vi "Configuration to String.vi"(8 "error in (no error)":errorcluster, 10 "Configuration":variant, 11 "Instrument":T2=enum."Switching Matrix") -> (0 "error out":errorcluster, 2 "Instrument Configuration":T1={"Instrument"=enum."Switching Matrix", "Configuration"="Test Configuration"})   [LabVIEW 2014]
uses:
  Measurements/Instrument Sequence/Hardware Configuration.ctl
  Hardware Control/Spectrometer/Spectrometer Config.ctl
  Hardware Control/Spectrometer/Laser Settings.ctl
  Hardware Control/Spectrometer/Laser.ctl
  Hardware Control/Spectrometer/Filter.ctl
  Hardware Control/Spectrometer/Grating Detector Settings.ctl
  Hardware Control/Spectrometer/Grating.ctl
  Hardware Control/Spectrometer/Detector.ctl
  Hardware Control/Spectrometer/Acquisition Settings.ctl
  Hardware Control/Switches and Mirrors/SwitchesMirrors Config.ctl
  Hardware Control/Switches and Mirrors/SwitchesMirrors Status.ctl
  Hardware Control/Stress Control/StressControl Config.ctl
  Hardware Control/Parameter Analyzer/Parameter Analyzer Config.ctl
  Hardware Control/Parameter Analyzer/Parameter Analyzer Integration Parameters.ctl
  Hardware Control/Parameter Analyzer/Parameter Analyzer SMU Sweeping.ctl
  Hardware Control/Parameter Analyzer/Parameter Analyzer Sweep Spacing.ctl
  Hardware Control/Parameter Analyzer/Parameter Analyzer SMU Range.ctl
  Hardware Control/Parameter Analyzer/Parameter Analyzer SMU Sampling.ctl
  Hardware Control/Parameter Analyzer/Parameter Analyzer Sampling Parameters.ctl
  Hardware Control/Parameter Analyzer/Parameter Analyzer Stop Sampling Conditions.ctl
  Hardware Control/Switching Matrix/Switching Matrix Config.ctl
  Measurements/Save Data/SaveData Workspace Info.ctl
  Measurements/Instrument Sequence/Instrument List.ctl
  Measurements/Save Data/SaveData Instrument Configuration.ctl
panel:
  in  "Hardware Configuration":T3={"Optical Spectrometer"={"Laser Settings"={"Laser Wavelength"=enum."784 nm", "Neutral Density Filter"=enum."50%"}, "Spectrometer Settings"={"Confocal Hole Size (µm)"=150.0, "Grating"=2, "Detector"=enum."InGaAs Array"}, "Acquisition Settings"={"Acquisition Mode"=enum."Single Window", "Spectal Position (nm)"=632.84, "From (nm)"=632.84, "To (nm)"=1.0, "Integration Time (s)"=3.0, "Number of Accumulations"=3, "AutoScanning"=FALSE, "Spike Removal"=FALSE}, "Path"=path ""}, "Switches & Mirrors"={"Relay VISA Session"="COM1", "Switches"={"Laser"=FALSE, "Video"=FALSE}, "Delays (ms)"={"Laser"=500, "Video"=1500}}, "StressControl"={"Stress Control VISA Session"="COM4", "Axis"=1, "Motion"=0, "Destination (°)"=0.0, "Speed (°/s)"=4.0, "Position (°)"=0.0}, "Parameter Analizer"={"Parameter Analyzer VISA Session"="GPIB0::27::INSTR", "Sweeping Time Parameters"={"Integration Time"=0, "Short Integration Time (s)"=0.00192, "Long Integration Time (s)"=0.02, "Wait Time Parameter"=1.0}, "Acquisition Mode"=enum."Sweeping Mode", "Status Polling Time (ms)"=1000, "Comment"="", "SMU 1 - Sweeping"={"Start / Offset"=0.0, "Stop / Ratio"=10.0, "Step \n(linear only)"=0.01, "Compliance"=0.1, "Power \nCompliance"=0.0, "Mode"=0, "Function"=1, "Sweep Mode"=FALSE}, "SMU 2 - Sweeping"={"Start / Offset"=0.0, "Stop / Ratio"=1.0, "Step \n(linear only)"=0.01, "Compliance"=10.0, "Power \nCompliance"=0.0, "Mode"=1, "Function"=4, "Sweep Mode"=FALSE}, "SMU 3 - Sweeping"={"Start / Offset"=0.0, "Stop / Ratio"=1.0, "Step \n(linear only)"=0.01, "Compliance"=10.0, "Power \nCompliance"=0.0, "Mode"=1, "Function"=4, "Sweep Mode"=FALSE}, "SMU 4 - Sweeping"={"Start / Offset"=0.0, "Stop / Ratio"=1.0, "Step \n(linear only)"=0.01, "Compliance"=0.1, "Power \nCompliance"=0.0, "Mode"=0, "Function"=4, "Sweep Mode"=FALSE}, "Sweep Spacing"=0, "Range"=0, "SMU1 - Sampling"={"Source"=10.0, "Compliance"=0.01, "Mode"=0, "Function"=FALSE}, "SMU2 - Sampling"={"Source"=0.0, "Compliance"=10.0, "Mode"=1, "Function"=FALSE}, "SMU3 - Sampling"={"Source"=0.0, "Compliance"=10.0, "Mode"=1, "Function"=FALSE}, "SMU4 - Sampling"={"Source"=0.0, "Compliance"=0.01, "Mode"=0, "Function"=FALSE}, "Sampling Time Parameters"={"Initial Interval (s)"=0.1, "Number of Samples"=60, "Total Sampling Time (s)"=10.0, "Hold Time (s)"=0.0, "Sampling Mode"=0, "Sampling Time"=0}, "Stop Condition"={"Enable Delay (s)"=0.0, "Name"="", "Threshold"=0.0, "num. of events"=1, "Event"=0, "Stop Condition Enable"=FALSE}}, "Switching Matrix"={"Switching Matrix VISA Session"="GPIB0::18::INSTR", "Connections"=[{"Connections"=[TRUE, FALSE, FALSE, FALSE, FALSE, FALSE, FALSE, FALSE, FALSE, FALSE, FALSE, FALSE], "Connection Type"=enum."Make - Break"}, {"Connections"=[FALSE, TRUE, FALSE, FALSE, FALSE, FALSE, FALSE, FALSE, FALSE, FALSE, FALSE, FALSE], "Connection Type"=enum."Make - Break"}, {"Connections"=[FALSE, FALSE, TRUE, FALSE, FALSE, FALSE, FALSE, FALSE, FALSE, FALSE, FALSE, FALSE], "Connection Type"=enum."Make - Break"}, {"Connections"=[FALSE, FALSE, FALSE, TRUE, FALSE, FALSE, FALSE, FALSE, FALSE, FALSE, FALSE, FALSE], "Connection Type"=enum."Make - Break"}, {"Connections"=[FALSE, FALSE, FALSE, FALSE, TRUE, TRUE, TRUE, TRUE, TRUE, TRUE, TRUE, TRUE], "Connection Type"=enum."Make - Break"}, {"Connections"=[FALSE, FALSE, FALSE, FALSE, FALSE, FALSE, FALSE, FALSE, FALSE, FALSE, FALSE, FALSE], "Connection Type"=enum."Disconnected"}, {"Connections"=[FALSE, FALSE, FALSE, FALSE, FALSE, FALSE, FALSE, FALSE, FALSE, FALSE, FALSE, FALSE], "Connection Type"=enum."Disconnected"}, {"Connections"=[FALSE, FALSE, FALSE, FALSE, FALSE, FALSE, FALSE, FALSE, FALSE, FALSE, FALSE, FALSE], "Connection Type"=enum."Disconnected"}]}, "Electrical Measurement"={"Measurement Type"=enum."Four Probe", "Sweep Mode"=FALSE, "Force Mode"=enum."Voltage", "Maximum Force"=0.15, "Step Size"=0.001, "Compliance"=0.001, "Power Compliance"=0.0, "Integration Time (s)"=0.02}, "Workspace Info"={"Device Name"="test", "Device Info"="test", "Path"=path "C:/Users/gio/Desktop/test Python2Workspace/python2workspace_test.pmat"}, "AutoFocus Status"={"Update Refnums"=FALSE, "Allocate Image Memory"=FALSE, "Set Match Criteria"=FALSE, "Link Stage & Camera"=FALSE, "Set Target"=FALSE, "Find Target"=FALSE}} {"Electrical Measurement"."Integration Time (s)" min=0.02 max=2.0 scale=8e-05..2.0; "Electrical Measurement"."Power Compliance" format="%^.2e"; "Electrical Measurement"."Compliance" format="%^.2e"; "Electrical Measurement"."Step Size" format="%^.4e"; "Electrical Measurement"."Maximum Force" format="%^.4e"; "Parameter Analizer"."Stop Condition"."Event" items=["Value > Threshold", "Value < Threshold", "| Value | > | Threshold |", "| Value | < | Threshold |"]; "Parameter Analizer"."Stop Condition"."Threshold" format="%^.2e"; "Parameter Analizer"."Stop Condition"."Enable Delay (s)" format="%.1f"; "Parameter Analizer"."Sampling Time Parameters"."Sampling Time" items=["Auto (linear only)", "No Limit", "Set Limit"]; "Parameter Analizer"."Sampling Time Parameters"."Sampling Mode" items=["Linear", "Log10", "Log25", "Log50", "Thinned Out"]; "Parameter Analizer"."Sampling Time Parameters"."Hold Time (s)" format="%.4f"; "Parameter Analizer"."Sampling Time Parameters"."Total Sampling Time (s)" format="%.1f"; "Parameter Analizer"."Sampling Time Parameters"."Initial Interval (s)" format="%^.3e"; "Parameter Analizer"."SMU 4 - Sweeping"."Function" items=["Disabled", "Var 1", "Var 2", "Var 1'", "Constant"]; "Parameter Analizer"."SMU 4 - Sweeping"."Mode" items=["V", "I", "V pulse", "I  pulse", "Common"]; "Parameter Analizer"."SMU 4 - Sweeping"."Power \nCompliance" format="%^.2e"; "Parameter Analizer"."SMU 4 - Sweeping"."Compliance" format="%^.2e"; "Parameter Analizer"."SMU 4 - Sweeping"."Step \n(linear only)" format="%^.4e"; "Parameter Analizer"."SMU 4 - Sweeping"."Stop / Ratio" format="%^.4e"; "Parameter Analizer"."SMU 4 - Sweeping"."Start / Offset" format="%^.4e"; "Parameter Analizer"."SMU 3 - Sweeping"."Function" items=["Disabled", "Var 1", "Var 2", "Var 1'", "Constant"]; "Parameter Analizer"."SMU 3 - Sweeping"."Mode" items=["V", "I", "V pulse", "I  pulse", "Common"]; "Parameter Analizer"."SMU 3 - Sweeping"."Power \nCompliance" format="%^.2e"; "Parameter Analizer"."SMU 3 - Sweeping"."Compliance" format="%^.2e"; "Parameter Analizer"."SMU 3 - Sweeping"."Step \n(linear only)" format="%^.4e"; "Parameter Analizer"."SMU 3 - Sweeping"."Stop / Ratio" format="%^.4e"; "Parameter Analizer"."SMU 3 - Sweeping"."Start / Offset" format="%^.4e"; "Parameter Analizer"."SMU 2 - Sweeping"."Function" items=["Disabled", "Var 1", "Var 2", "Var 1'", "Constant"]; "Parameter Analizer"."SMU 2 - Sweeping"."Mode" items=["V", "I", "V pulse", "I  pulse", "Common"]; "Parameter Analizer"."SMU 2 - Sweeping"."Power \nCompliance" format="%^.2e"; "Parameter Analizer"."SMU 2 - Sweeping"."Compliance" format="%^.2e"; "Parameter Analizer"."SMU 2 - Sweeping"."Step \n(linear only)" format="%^.4e"; "Parameter Analizer"."SMU 2 - Sweeping"."Stop / Ratio" format="%^.4e"; "Parameter Analizer"."SMU 2 - Sweeping"."Start / Offset" format="%^.4e"; "Parameter Analizer"."SMU 1 - Sweeping"."Function" items=["Disabled", "Var 1", "Var 2", "Var 1'", "Constant"]; "Parameter Analizer"."SMU 1 - Sweeping"."Mode" items=["V", "I", "V pulse", "I  pulse", "Common"]; "Parameter Analizer"."SMU 1 - Sweeping"."Power \nCompliance" format="%^.2e"; "Parameter Analizer"."SMU 1 - Sweeping"."Compliance" format="%^.2e"; "Parameter Analizer"."SMU 1 - Sweeping"."Step \n(linear only)" format="%^.4e"; "Parameter Analizer"."SMU 1 - Sweeping"."Stop / Ratio" format="%^.4e"; "Parameter Analizer"."SMU 1 - Sweeping"."Start / Offset" format="%^.4e"; "Parameter Analizer"."Sweeping Time Parameters"."Long Integration Time (s)" scale=0.02..2.0; "Parameter Analizer"."Sweeping Time Parameters"."Short Integration Time (s)" scale=8e-05..0.00192; "Parameter Analizer"."Sweeping Time Parameters"."Integration Time" items=["Short", "Long"]; "Parameter Analizer"."Sweeping Time Parameters"."Wait Time Parameter" format="%.1f"; "Parameter Analizer"."SMU4 - Sampling"."Mode" items=["V", "I", "Common"]; "Parameter Analizer"."SMU4 - Sampling"."Compliance" format="%^.2e"; "Parameter Analizer"."SMU4 - Sampling"."Source" format="%^.3e"; "Parameter Analizer"."SMU3 - Sampling"."Mode" items=["V", "I", "Common"]; "Parameter Analizer"."SMU3 - Sampling"."Compliance" format="%^.2e"; "Parameter Analizer"."SMU3 - Sampling"."Source" format="%^.3e"; "Parameter Analizer"."SMU2 - Sampling"."Mode" items=["V", "I", "Common"]; "Parameter Analizer"."SMU2 - Sampling"."Compliance" format="%^.2e"; "Parameter Analizer"."SMU2 - Sampling"."Source" format="%^.3e"; "Parameter Analizer"."SMU1 - Sampling"."Mode" items=["V", "I", "Common"]; "Parameter Analizer"."SMU1 - Sampling"."Compliance" format="%^.2e"; "Parameter Analizer"."SMU1 - Sampling"."Source" format="%^.3e"; "Parameter Analizer"."Range" items=["auto", "fixed", "limited"]; "Parameter Analizer"."Sweep Spacing" items=["linear", "log 10", "log 25", "log 50"]; "StressControl"."Axis" min=1 max=3; "StressControl"."Position (°)" format="%.6g"; "StressControl"."Speed (°/s)" min=0.0 max=4.0 format="%.6f"; "StressControl"."Destination (°)" min=-2000000000.0 max=2000000000.0 format="%.6f"; "StressControl"."Motion" items=["Absolute", "Relative"]; "Optical Spectrometer"."Spectrometer Settings"."Grating" items=["1800 l/mm", "150 l/mm"]}
  # "LICENSED MATERIALS – PROPERTY OF IBM\nCopyright IBM Corp. 2016,\nALL RIGHTS RESERVED"
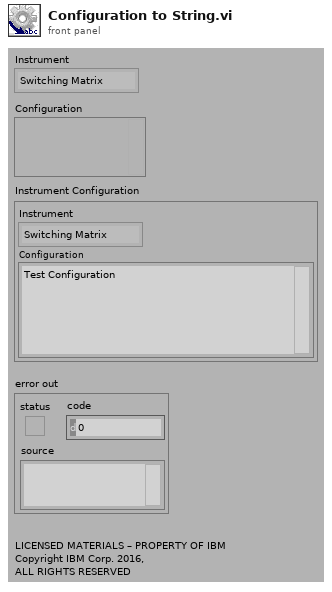
[diagram p1: front panel]
types:
  T1 = typedef "SaveData Instrument Configuration.ctl" = cluster{"Instrument":T2, "Configuration":string}
  T2 = typedef "Instrument List.ctl" = enum32{"Unknown Instrument", "Switching Matrix", "Parameter Analyzer", "Optical Spectrometer", "Optoelectronic", "Autofocus"}
  T3 = typedef "Hardware Configuration.ctl" = cluster{"Optical Spectrometer":T4, "Switches & Mirrors":T12, "StressControl":T14, "Parameter Analizer":T15, "Switching Matrix":T23, "Electrical Measurement":cluster{"Measurement Type":enum32{"Four Probe", "Two Probe"}, "Sweep Mode":bool, "Force Mode":enum32{"Voltage", "Current"}, "Maximum Force":dbl, "Step Size":dbl, "Compliance":dbl, "Power Compliance":dbl, "Integration Time (s)":dbl}, "Workspace Info":T24, "AutoFocus Status":cluster{"Update Refnums":bool, "Allocate Image Memory":bool, "Set Match Criteria":bool, "Link Stage & Camera":bool, "Set Target":bool, "Find Target":bool}}
  T4 = typedef "Spectrometer Config.ctl" = cluster{"Laser Settings":T5, "Spectrometer Settings":T8, "Acquisition Settings":T11, "Path":path}
  T5 = typedef "Laser Settings.ctl" = cluster{"Laser Wavelength":T6, "Neutral Density Filter":T7}
  T6 = typedef "Laser.ctl" = enum16{"633 nm", "784 nm", "532 nm", "365 nm"}
  T7 = typedef "Filter.ctl" = enum16{"100%", "50%", "25%", "10%", "1%", "0.1%", "0.01%"}
  T8 = typedef "Grating Detector Settings.ctl" = cluster{"Confocal Hole Size (µm)":dbl, "Grating":T9, "Detector":T10}
  T9 = typedef "Grating.ctl" = u16
  T10 = typedef "Detector.ctl" = enum16{"InGaAs Array", "Silicon CCD"}
  T11 = typedef "Acquisition Settings.ctl" = cluster{"Acquisition Mode":enum16{"Single Window", "Multi-Window"}, "Spectal Position (nm)":dbl, "From (nm)":dbl, "To (nm)":dbl, "Integration Time (s)":dbl, "Number of Accumulations":i32, "AutoScanning":bool, "Spike Removal":bool}
  T12 = typedef "SwitchesMirrors Config.ctl" = cluster{"Relay VISA Session":refnum<visa-resource-name>, "Switches":T13, "Delays (ms)":cluster{"Laser":u32, "Video":u32}}
  T13 = typedef "SwitchesMirrors Status.ctl" = cluster{"Laser":bool, "Video":bool}
  T14 = typedef "StressControl Config.ctl" = cluster{"Stress Control VISA Session":refnum<visa-resource-name>, "Axis":i32, "Motion":u16, "Destination (°)":dbl, "Speed (°/s)":dbl, "Position (°)":dbl}
  T15 = typedef "Parameter Analyzer Config.ctl" = cluster{"Parameter Analyzer VISA Session":refnum<visa-resource-name>, "Sweeping Time Parameters":T16, "Acquisition Mode":enum32{"Sweeping Mode", "Sampling Mode"}, "Status Polling Time (ms)":u32, "Comment":string, "SMU 1 - Sweeping":T17, "SMU 2 - Sweeping":T17, "SMU 3 - Sweeping":T17, "SMU 4 - Sweeping":T17, "Sweep Spacing":T18, "Range":T19, "SMU1 - Sampling":T20, "SMU2 - Sampling":T20, "SMU3 - Sampling":T20, "SMU4 - Sampling":T20, "Sampling Time Parameters":T21, "Stop Condition":T22}
  T16 = typedef "Parameter Analyzer Integration Parameters.ctl" = cluster{"Integration Time":u32, "Short Integration Time (s)":dbl, "Long Integration Time (s)":dbl, "Wait Time Parameter":dbl}
  T17 = typedef "Parameter Analyzer SMU Sweeping.ctl" = cluster{"Start / Offset":dbl, "Stop / Ratio":dbl, "Step \n(linear only)":dbl, "Compliance":dbl, "Power \nCompliance":dbl, "Mode":u32, "Function":i32, "Sweep Mode":bool}
  T18 = typedef "Parameter Analyzer Sweep Spacing.ctl" = u16
  T19 = typedef "Parameter Analyzer SMU Range.ctl" = u16
  T20 = typedef "Parameter Analyzer SMU Sampling.ctl" = cluster{"Source":dbl, "Compliance":dbl, "Mode":u32, "Function":bool}
  T21 = typedef "Parameter Analyzer Sampling Parameters.ctl" = cluster{"Initial Interval (s)":dbl, "Number of Samples":i32, "Total Sampling Time (s)":dbl, "Hold Time (s)":dbl, "Sampling Mode":i32, "Sampling Time":i32}
  T22 = typedef "Parameter Analyzer Stop Sampling Conditions.ctl" = cluster{"Enable Delay (s)":dbl, "Name":string, "Threshold":dbl, "num. of events":i32, "Event":i32, "Stop Condition Enable":bool}
  T23 = typedef "Switching Matrix Config.ctl" = cluster{"Switching Matrix VISA Session":refnum<visa-resource-name>, "Connections":cluster{"Connections":bool[], "Connection Type":enum16{"Disconnected", "Make - Break", "Break - Make"}}[]}
  T24 = typedef "SaveData Workspace Info.ctl" = cluster{"Device Name":string, "Device Info":string, "Path":path}
  T25 = cluster{"Connections":bool[], "Connection Type":enum16{"Disconnected", "Make - Break", "Break - Make"}}[]
  T26 = enum16{"Disconnected", "Make - Break", "Break - Make"}
  T27 = cluster{"Optical Spectrometer":T4, "Switches":T13}
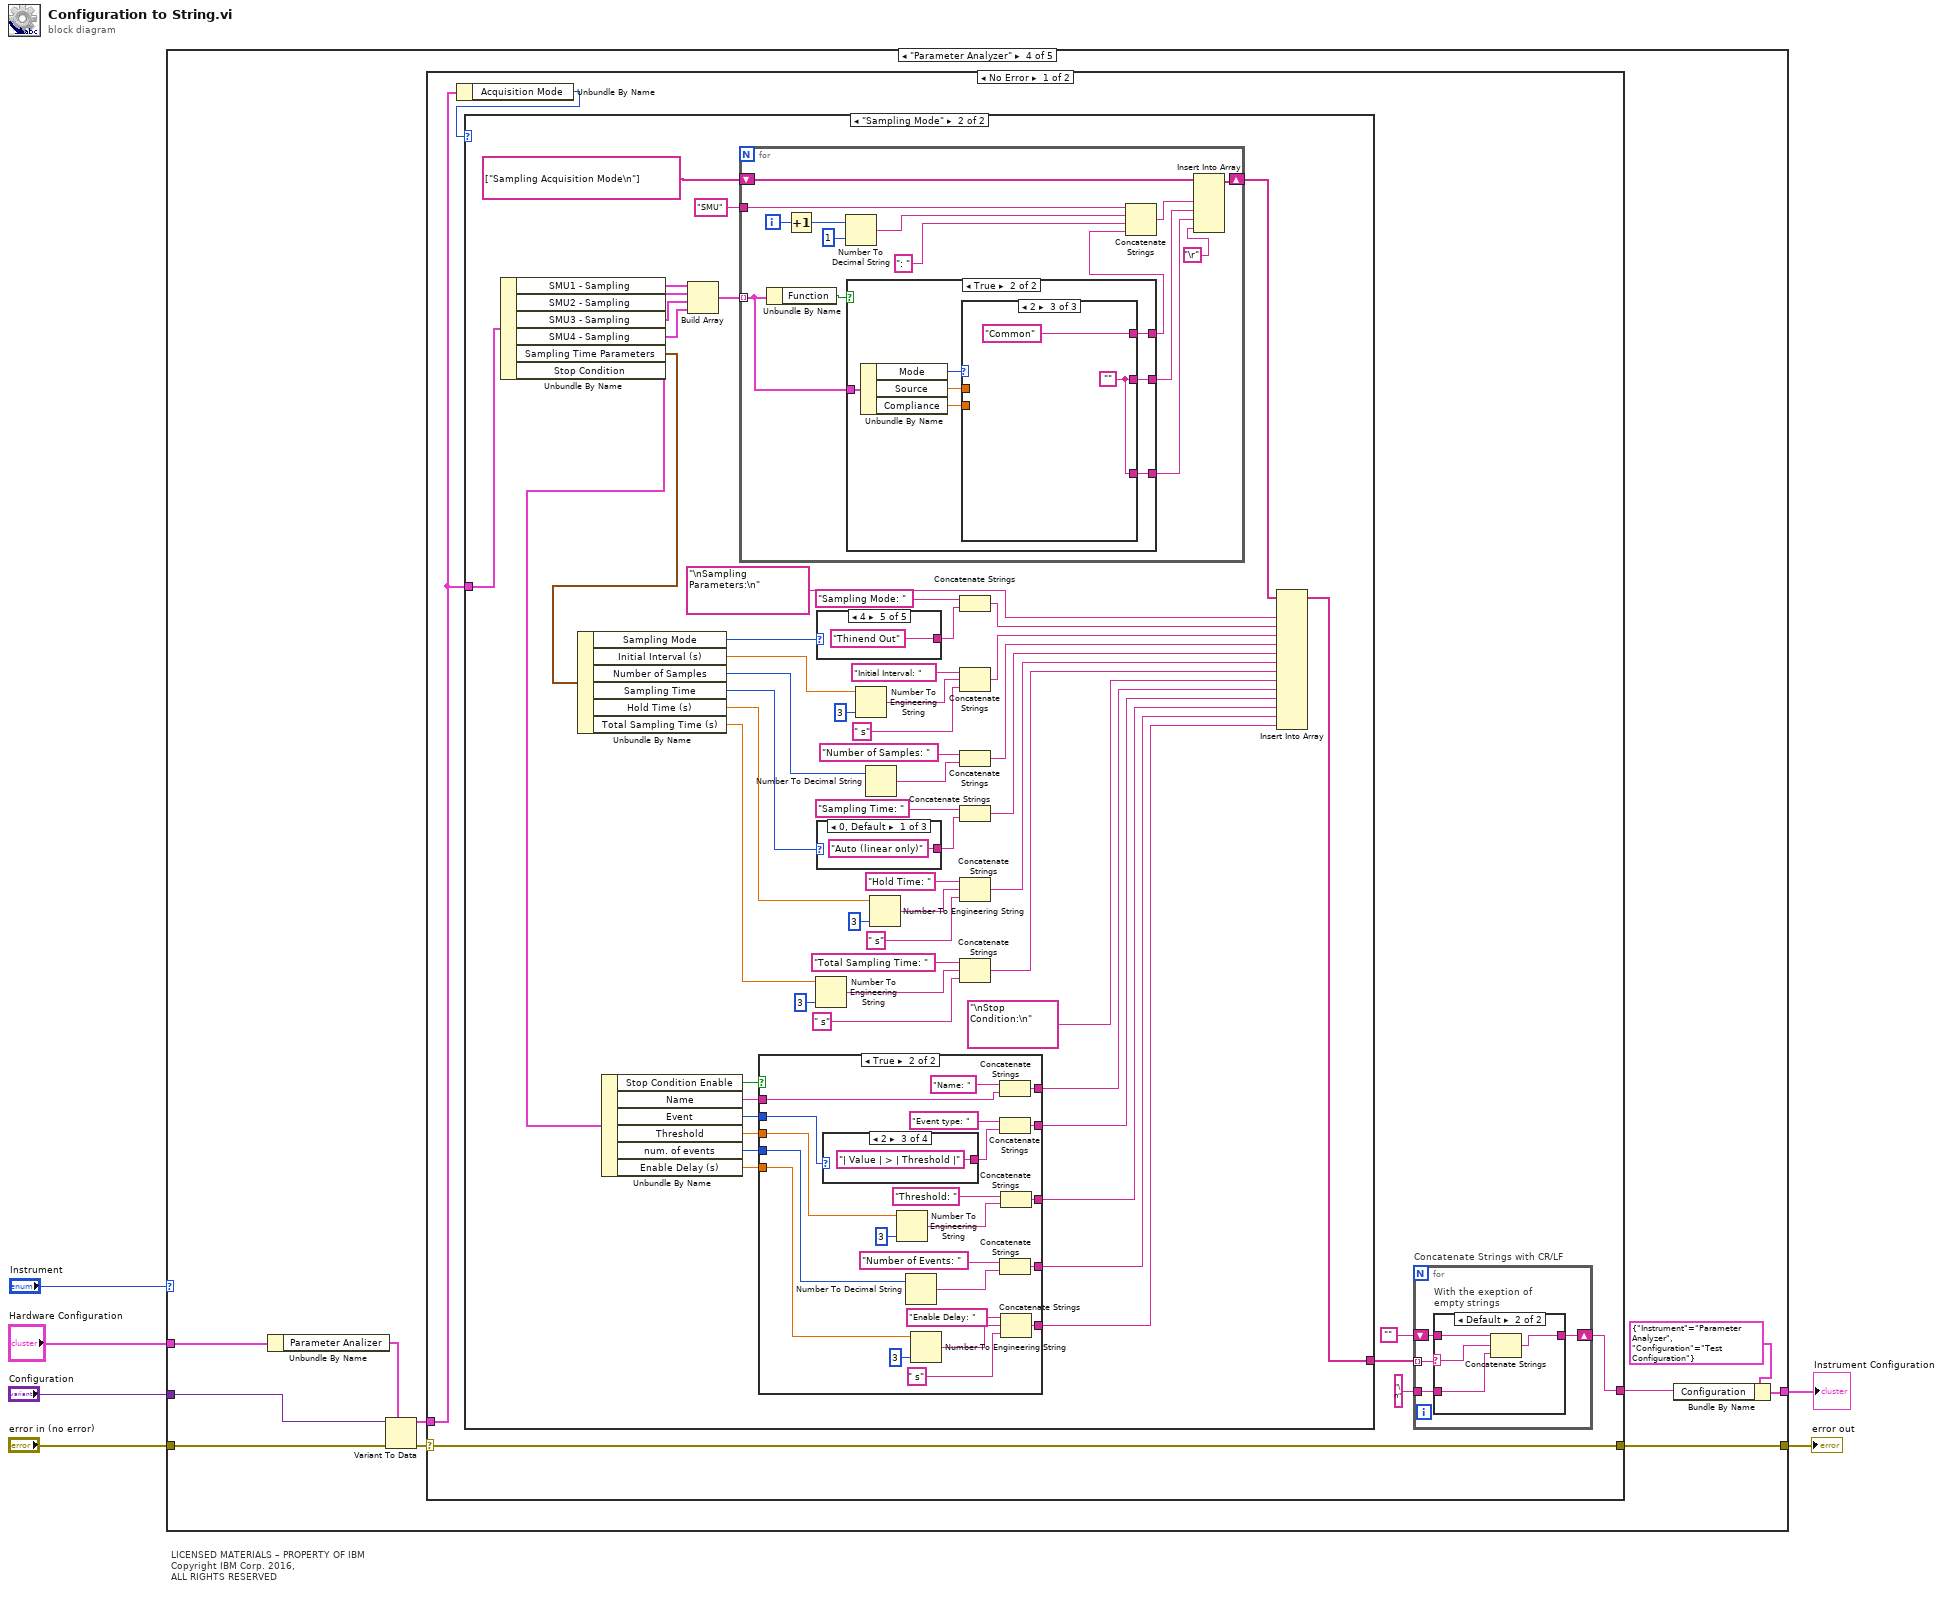
[diagram p0: block diagram]
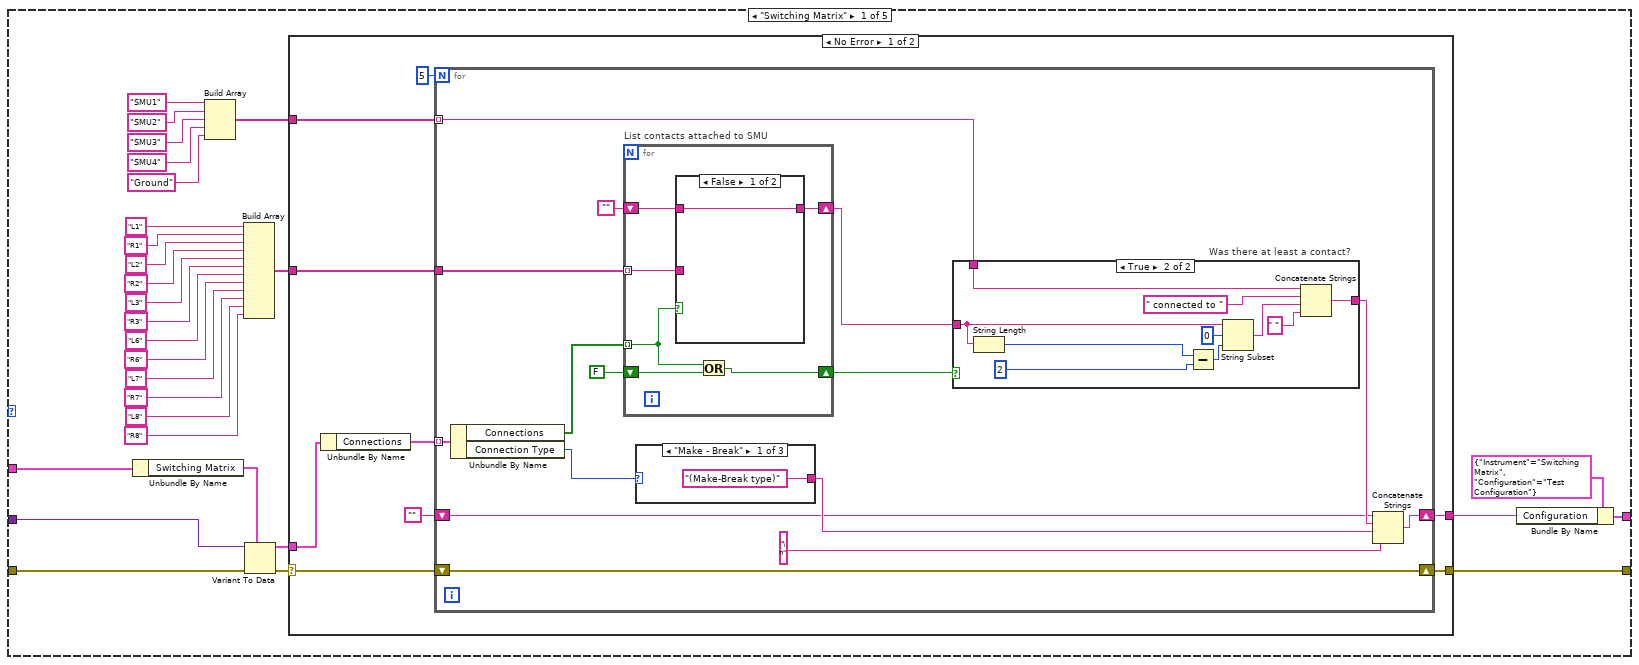
[diagram p2: hidden frame]
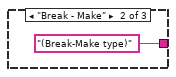
[diagram p3: hidden frame]
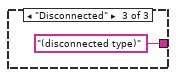
[diagram p4: hidden frame]
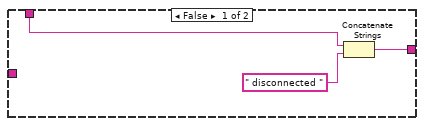
[diagram p5: hidden frame]
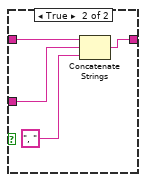
[diagram p6: hidden frame]
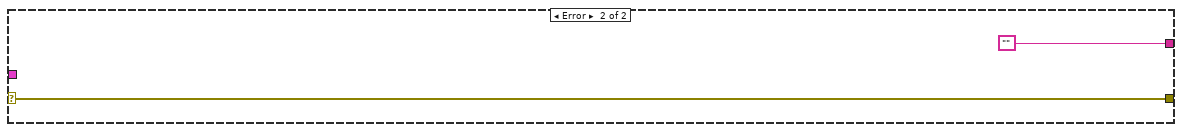
[diagram p7: hidden frame]
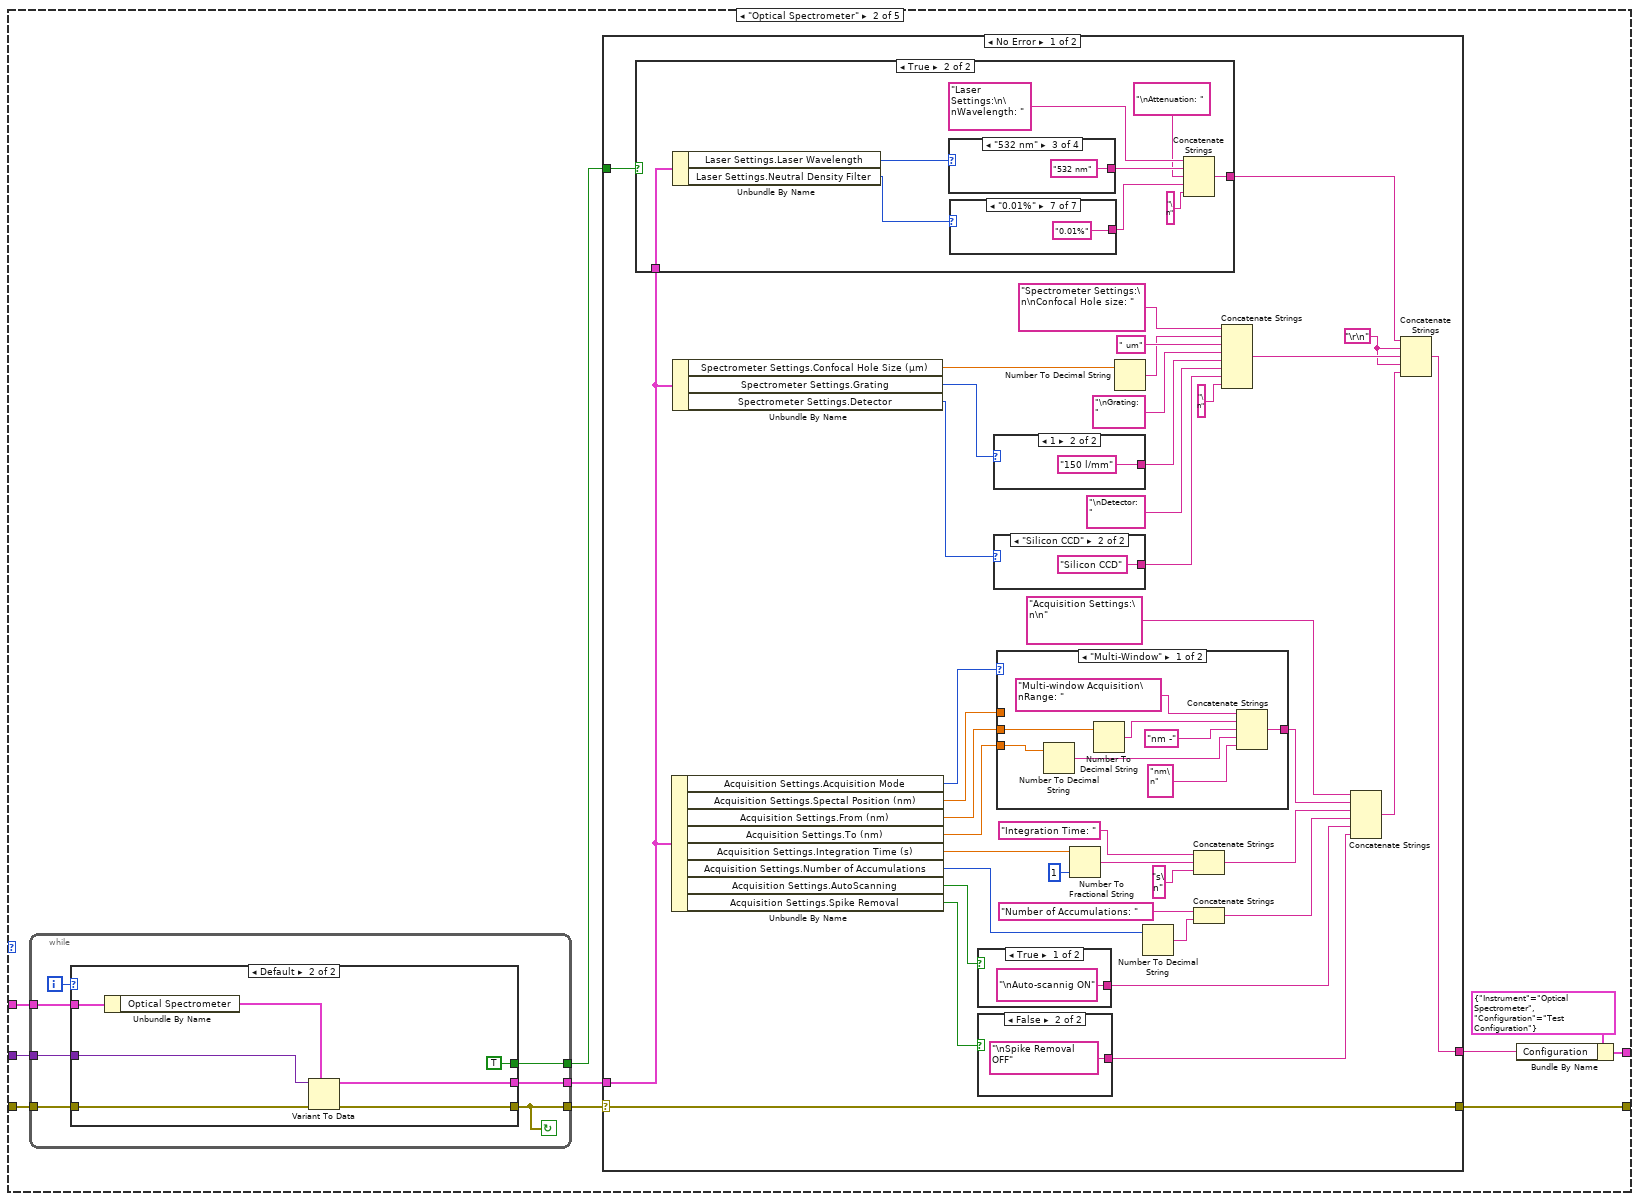
[diagram p8: hidden frame]
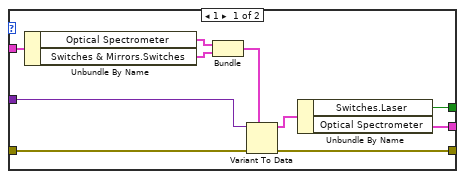
[diagram p9: hidden frame]
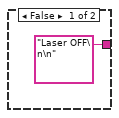
[diagram p10: hidden frame]
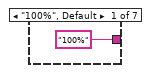
[diagram p11: hidden frame]
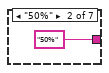
[diagram p12: hidden frame]
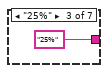
[diagram p13: hidden frame]
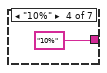
[diagram p14: hidden frame]
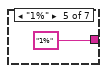
[diagram p15: hidden frame]
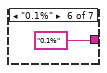
[diagram p16: hidden frame]
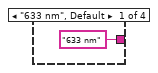
[diagram p17: hidden frame]
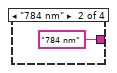
[diagram p18: hidden frame]
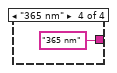
[diagram p19: hidden frame]
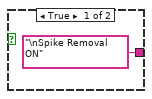
[diagram p20: hidden frame]
diagram:
  # "LICENSED MATERIALS – PROPERTY OF IBM\nCopyright IBM Corp. 2016,\nALL RIGHTS RESERVED"
  n1 = case shown="\"Parameter Analyzer\"" "Instrument" {
    tunnel: "Hardware Configuration" -> [w35 w98 _ w215 _]
    tunnel: "error in (no error)" -> [w34 w97 w207 w217 w570]
    tunnel: [w30 w96 w207 w211 w571] -> w2
    tunnel: "Configuration" -> [w33 w90 _ w216 _]
    tunnel: [w7 w93 T1 {"Instrument"=enum."Autofocus", "Configuration"="Autofocus ON"} ("Instrument Configuration 2") w208 T1 {"Instrument"=enum."Unknown Instrument", "Configuration"=""} ("Instrument Configuration 2")] -> w1
    frame "Switching Matrix" {
      n2 = Unbundle By Name(w35) -> ("Switching Matrix"=w32:T23)
      n3 = Build Array("SMU1", "SMU2", "SMU3", "SMU4", "Ground") -> (w24:string[])
      n4 = Build Array("L1", "R1", "L2", "R2", "L3", "R3", "L6", "R6", "L7", "R7", "L8", "R8") -> (w11:string[])
      n5 = Variant To Data(error in=w34, type=w32, Variant=w33) -> (data=w31:T23, error out=w10:errorcluster)
      n6 = case shown="No Error" w10 {
        selector: w10 -> [w36 w88]
        tunnel: w31 -> [w44 _]
        tunnel: [w42 w88] -> w30
        tunnel: w24 -> [w41 _]
        tunnel: w11 -> [w39 _]
        tunnel: [w37 ""] -> w8
        frame No Error {
          n7 = Unbundle By Name(w44) -> ("Connections"=w43:T25)
          n8 = for {
            N: 5 -> [_]
            tunnel: w43 -> [w58] mode=indexing
            shift-right: [w59] -> w42
            shift-left: w36 -> [w59]
            tunnel: w41 -> [w51] mode=indexing
            tunnel: w39 -> [w56]
            shift-right: [w45] -> w37
            shift-left: "" -> [w47]
            n9 = Unbundle By Name(w58) -> ("Connections"=w57:bool[], "Connection Type"=w50:T26)
            n10 = for "List contacts attached to SMU" {
              tunnel: w57 -> [w78] mode=indexing
              tunnel: w56 -> [w80] mode=indexing
              shift-right: [w79] -> w55
              shift-left: "" -> [w81]
              shift-right: [w76] -> w53
              shift-left: FALSE -> [w77]
              n11 = case shown="False" w78 {
                tunnel: w81 -> [w82 w86]
                tunnel: w80 -> [_ w84]
                tunnel: [w82 w83] -> w79
                frame False {
                }
                frame True {
                  n12 = Concatenate Strings(w86, w84, ", ") -> (w83:string)
                }
              }
              n13 = Or(x=w78, y=w77) -> (x .or. y?=w76:bool)
            }
            n14 = case shown="\"Make - Break\"" w50 {
              tunnel: ["(Make-Break type)" "(Break-Make type)" "(disconnected type)"] -> w48
              frame "Make - Break" {
              }
              frame "Break - Make" {
              }
              frame "Disconnected" {
              }
            }
            n15 = case "Was there at least a contact?" shown="True" w53 {
              tunnel: w55 -> [_ w74]
              tunnel: [w63 w71] -> w49
              tunnel: w51 -> [w65 w70]
              frame False {
                n16 = Concatenate Strings(w65, " disconnected ") -> (w63:string)
              }
              frame True {
                n17 = String Length(string=w74) -> (length=w66:i32)
                n18 = Subtract(x=w66, y=2 ("length (rest)")) -> (x-y=w67:i32)
                n19 = String Subset(string=w74, offset (0)=0, length (rest)=w67) -> (substring=w73:string)
                n20 = Concatenate Strings(w70, " connected to ", w73, " ") -> (w71:string)
              }
            }
            n21 = Concatenate Strings(w47, w49, w48, "\n") -> (w45:string)
          }
        }
        frame Error {
        }
      }
      n22 = Bundle By Name(cluster=T1 {"Instrument"=enum."Switching Matrix", "Configuration"="Test Configuration"} ("Instrument Configuration 2"), "Configuration"=w8) -> (w7:T1)
    }
    frame "Optical Spectrometer" {
      n23 = while {
        tunnel: w98 -> [w105]
        tunnel: w97 -> [w104]
        tunnel: [w103] -> w92
        tunnel: [w102] -> w91
        tunnel: w90 -> [w101]
        tunnel: [w99] -> w89
        i -> [w100]
        stop <- w99 continue-if-true
        n24 = case shown="Default" w100 {
          tunnel: w105 -> [w115 w122]
          tunnel: w104 -> [w114 w121]
          tunnel: [w111 w117] -> w103
          tunnel: [w110 TRUE ("Laser")] -> w102
          tunnel: w101 -> [w109 w120]
          tunnel: [w108 w119] -> w99
          frame 1 {
            n25 = Unbundle By Name(w115) -> ("Optical Spectrometer"=w107:T4, "Switches & Mirrors.Switches"=w106:T13)
            n26 = Bundle("Optical Spectrometer"=w107, "Switches"=w106) -> (w112:T27)  [unwired: 1 in]
            n27 = Variant To Data(error in=w114, type=w112, Variant=w109) -> (data=w113:T27, error out=w108:errorcluster)
            n28 = Unbundle By Name(w113) -> ("Switches.Laser"=w110:bool, "Optical Spectrometer"=w111:T4)
          }
          frame Default {
            n29 = Unbundle By Name(w122) -> ("Optical Spectrometer"=w118:T4)
            n30 = Variant To Data(error in=w121, type=w118, Variant=w120) -> (data=w117:T4, error out=w119:errorcluster)
          }
        }
      }
      n31 = case shown="No Error" w89 {
        selector: w89 -> [w161 w205]
        tunnel: w92 -> [w149 _]
        tunnel: [w161 w205] -> w96
        tunnel: [w127 ""] -> w94
        tunnel: w91 -> [w123 _]
        frame No Error {
          w124 = "\r\n"
          n32 = case shown="True" w123 {
            tunnel: w149 -> [_ w169]
            tunnel: ["Laser OFF\n\n" w168] -> w126
            frame False {
            }
            frame True {
              n33 = Unbundle By Name(w169) -> ("Laser Settings.Laser Wavelength"=w171:T6, "Laser Settings.Neutral Density Filter"=w170:T7)
              n34 = case shown="\"532 nm\"" w171 {
                tunnel: ["633 nm" "784 nm" "532 nm" "365 nm"] -> w166
                frame "633 nm", Default {
                }
                frame "784 nm" {
                }
                frame "532 nm" {
                }
                frame "365 nm" {
                }
              }
              n35 = case shown="\"0.01%\"" w170 {
                tunnel: ["100%" "50%" "25%" "10%" "1%" "0.1%" "0.01%"] -> w164
                frame "100%", Default {
                }
                frame "50%" {
                }
                frame "25%" {
                }
                frame "10%" {
                }
                frame "1%" {
                }
                frame "0.1%" {
                }
                frame "0.01%" {
                }
              }
              n36 = Concatenate Strings("Laser Settings:\n\nWavelength: ", w166, "\nAttenuation: ", w164, "\n" ("string")) -> (w168:string)
            }
          }
          n37 = Unbundle By Name(w149) -> ("Acquisition Settings.Acquisition Mode"=w147:enum16{"Single Window", "Multi-Window"}, "Acquisition Settings.Spectal Position (nm)"=w146:dbl, "Acquisition Settings.From (nm)"=w145:dbl, "Acquisition Settings.To (nm)"=w144:dbl, "Acquisition Settings.Integration Time (s)"=w141:dbl, "Acquisition Settings.Number of Accumulations"=w143:i32, "Acquisition Settings.AutoScanning"=w135:bool, "Acquisition Settings.Spike Removal"=w134:bool)
          n38 = Unbundle By Name(w149) -> ("Spectrometer Settings.Confocal Hole Size (µm)"=w160:dbl, "Spectrometer Settings.Grating"=w156:T9, "Spectrometer Settings.Detector"=w153:T10)
          n39 = case shown="True" w135 {
            tunnel: ["\nAuto-scannig ON" "\nAuto-scannig OFF"] -> w130
            frame True {
            }
            frame False {
            }
          }
          n40 = case shown="False" w134 {
            tunnel: ["\nSpike Removal ON" "\nSpike Removal OFF"] -> w129
            frame True {
            }
            frame False {
            }
          }
          n41 = case shown="1" w156 {
            tunnel: ["1800 l/mm" "150 l/mm"] -> w154
            frame 0, Default {
            }
            frame 1 {
            }
          }
          n42 = case shown="\"Silicon CCD\"" w153 {
            tunnel: ["InGaAs Array" "Silicon CCD"] -> w151
            frame "InGaAs Array", Default {
            }
            frame "Silicon CCD" {
            }
          }
          n43 = case shown="\"Multi-Window\"" w147 {
            tunnel: w146 -> [_ w195]
            tunnel: w145 -> [w193 _]
            tunnel: w144 -> [w194 _]
            tunnel: [w187 w196] -> w133
            frame "Multi-Window" {
              n44 = Number To Decimal String(number=w194) -> (decimal integer string=w189:string)  [unwired: 1 out]
              n45 = Number To Decimal String(number=w193) -> (decimal integer string=w191:string)  [unwired: 1 out]
              n46 = Concatenate Strings("Multi-window Acquisition\nRange: ", w191, "nm -", w189, "nm\n") -> (w187:string)
            }
            frame "Single Window" {
              n47 = Number To Decimal String(number=w195) -> (decimal integer string=w198:string)  [unwired: 1 out]
              n48 = Concatenate Strings("Single Acquisition\nSpectral Position: ", w198, "nm\n") -> (w196:string)
            }
          }
          n49 = Number To Fractional String(number=w141, precision (6)=i16 1) -> (F-format string=w139:string)  [unwired: 2 in]
          n50 = Number To Decimal String(number=w160) -> (decimal integer string=w158:string)  [unwired: 1 out]
          n51 = Number To Decimal String(number=w143) -> (decimal integer string=w136:string)  [unwired: 1 out]
          n52 = Concatenate Strings("Integration Time: ", w139, "s\n") -> (w132:string)
          n53 = Concatenate Strings("Number of Accumulations: ", w136) -> (w131:string)
          n54 = Concatenate Strings("Spectrometer Settings:\n\nConfocal Hole size: ", w158, " um" ("string"), "\nGrating: ", w154, "\nDetector: ", w151, "\n" ("string")) -> (w128:string)
          n55 = Concatenate Strings("Acquisition Settings:\n\n", w133, w132, w131, w130, w129) -> (w125:string)
          n56 = Concatenate Strings(w126, w124, w128, w124, w125) -> (w127:string)
        }
        frame Error {
        }
      }
      n57 = Bundle By Name(cluster=T1 {"Instrument"=enum."Optical Spectrometer", "Configuration"="Test Configuration"} ("Instrument Configuration 2"), "Configuration"=w94) -> (w93:T1)
    }
    frame "Autofocus" {
    }
    frame "Parameter Analyzer" {
      n58 = Unbundle By Name(w215) -> ("Parameter Analizer"=w214:T15)
      n59 = Variant To Data(error in=w217, type=w214, Variant=w216) -> (data=w213:T15, error out=w212:errorcluster)
      n60 = case shown="No Error" w212 {
        selector: w212 -> [w224 w567]
        tunnel: w213 -> [w220 _]
        tunnel: [w224 w567] -> w211
        tunnel: [w221 ""] -> w210
        frame No Error {
          n61 = Unbundle By Name(w220) -> ("Acquisition Mode"=w219:enum32{"Sweeping Mode", "Sampling Mode"})
          n62 = case shown="\"Sampling Mode\"" w219 {
            tunnel: w220 -> [w226 w461]
            tunnel: [w239 w427] -> w218
            frame "Sweeping Mode", Default {
              n63 = Unbundle By Name(w226) -> ("SMU 1 - Sweeping"=w249:T17, "SMU 2 - Sweeping"=w248:T17, "SMU 3 - Sweeping"=w247:T17, "SMU 4 - Sweeping"=w246:T17, "Sweep Spacing"=w255:T18, "Range"=w252:T19)
              n64 = Unbundle By Name(w226) -> ("Sweeping Time Parameters"=w227:T16)
              n65 = Build Array(w249, w248, w247, w246) -> (w244:T17[])
              n66 = for "Concatenate SMU settings" {
                tunnel: "SMU" -> [w288]
                tunnel: w244 -> [w263] mode=indexing
                shift-right: [w274] -> w242
                shift-left: string[] ["Sweeping Acquisition Mode\n"] -> [w273]
                i -> [w291]
                n67 = Unbundle By Name(w263) -> ("Power \nCompliance"=w276:dbl)
                n68 = Unbundle By Name(w263) -> ("Function"=w283:i32)
                n69 = Increment(x=w291) -> (x+1=w265:i32)
                n70 = Number To Decimal String(number=w265, width (-)=i16 1) -> (decimal integer string=w289:string)
                n71 = case shown="4" w283 {
                  tunnel: ["disabled" w298 w330 w364 w384] -> w282
                  tunnel: [w294 w315 w348 "" w389] -> w270
                  tunnel: [w294 w302 w340 w367 w386] -> w269
                  tunnel: [w294 w301 w333 w366 w389] -> w268
                  tunnel: w263 -> [_ w300 w331 w362 w385]
                  frame 0, Default {
                    w294 = ""
                  }
                  frame 1 {
                    n72 = Unbundle By Name(w300) -> ("Mode"=w297:u32)
                    n73 = Unbundle By Name(w300) -> ("Sweep Mode"=w316:bool)
                    n74 = case shown="0" w297 {
                      tunnel: ["Common" "Voltage Source " "Current Source " "Pulsed Voltage Source " "Pulsed Current Source "] -> w296
                      frame 4, Default {
                      }
                      frame 0 {
                      }
                      frame 1 {
                      }
                      frame 2 {
                      }
                      frame 3 {
                      }
                    }
                    n75 = Unbundle By Name(w300) -> ("Start / Offset"=w313:dbl)
                    n76 = Unbundle By Name(w300) -> ("Stop / Ratio"=w304:dbl)
                    n77 = Unbundle By Name(w300) -> ("Mode"=w312:u32)
                    n78 = Unbundle By Name(w300) -> ("Mode"=w305:u32)
                    n79 = case shown="True" w316 {
                      tunnel: ["Double Sweep" "Single Sweep"] -> w315
                      frame True {
                      }
                      frame False {
                      }
                    }
                    n80 = case shown="0, 2, Default" w312 {
                      tunnel: [" V" " A"] -> w309
                      frame 0, 2, Default {
                      }
                      frame 1, 3 {
                      }
                    }
                    n81 = case shown="0, 2, Default" w305 {
                      tunnel: [" V" " A"] -> w308
                      frame 0, 2, Default {
                      }
                      frame 1, 3 {
                      }
                    }
                    n82 = Number To Engineering String(2:i16 3 ("precision (6)"), 4:w313) -> (0:w310:string)  [unwired: 2 out]
                    n83 = Number To Engineering String(2:i16 3 ("precision (6)"), 4:w304) -> (0:w307:string)  [unwired: 2 out]
                    n84 = Concatenate Strings(w296, "[var 1]") -> (w298:string)
                    n85 = Concatenate Strings("Minimum Value: ", w310, w309) -> (w302:string)
                    n86 = Concatenate Strings("Maximum Value: ", w307, w308) -> (w301:string)
                  }
                  frame 2 {
                    n87 = Unbundle By Name(w331) -> ("Sweep Mode"=w347:bool)
                    n88 = Unbundle By Name(w331) -> ("Mode"=w329:u32)
                    n89 = Unbundle By Name(w331) -> ("Start / Offset"=w345:dbl)
                    n90 = case shown="3" w329 {
                      tunnel: ["Common" "Voltage Source " "Current Source " "Pulsed Voltage Source " "Pulsed Current Source "] -> w328
                      frame 4, Default {
                      }
                      frame 0 {
                      }
                      frame 1 {
                      }
                      frame 2 {
                      }
                      frame 3 {
                      }
                    }
                    n91 = Unbundle By Name(w331) -> ("Stop / Ratio"=w335:dbl)
                    n92 = Unbundle By Name(w331) -> ("Mode"=w344:u32)
                    n93 = Unbundle By Name(w331) -> ("Mode"=w336:u32)
                    n94 = case shown="True" w347 {
                      tunnel: ["Double Sweep" "Single Sweep"] -> w348
                      frame True {
                      }
                      frame False {
                      }
                    }
                    n95 = case shown="0, 2, Default" w344 {
                      tunnel: [" V" " A"] -> w341
                      frame 0, 2, Default {
                      }
                      frame 1, 3 {
                      }
                    }
                    n96 = case shown="0, 2, Default" w336 {
                      tunnel: [" V" " A"] -> w339
                      frame 0, 2, Default {
                      }
                      frame 1, 3 {
                      }
                    }
                    n97 = Number To Engineering String(2:i16 3 ("precision (6)"), 4:w345) -> (0:w342:string)  [unwired: 2 out]
                    n98 = Number To Engineering String(2:i16 3 ("precision (6)"), 4:w335) -> (0:w338:string)  [unwired: 2 out]
                    n99 = Concatenate Strings(w328, "[var 2]") -> (w330:string)
                    n100 = Concatenate Strings("Minimum Value: ", w342, w341) -> (w340:string)
                    n101 = Concatenate Strings("Maximum Value: ", w338, w339) -> (w333:string)
                  }
                  frame 3 {
                    n102 = Unbundle By Name(w362) -> ("Mode"=w361:u32)
                    n103 = Unbundle By Name(w362) -> ("Start / Offset"=w374:dbl)
                    n104 = Unbundle By Name(w362) -> ("Stop / Ratio"=w369:dbl)
                    n105 = case shown="3" w361 {
                      tunnel: ["Common" "Voltage Source " "Current Source " "Pulsed Voltage Source " "Pulsed Current Source "] -> w360
                      frame 4, Default {
                      }
                      frame 0 {
                      }
                      frame 1 {
                      }
                      frame 2 {
                      }
                      frame 3 {
                      }
                    }
                    n106 = Number To Engineering String(2:i16 3 ("precision (6)"), 4:w374) -> (0:w372:string)  [unwired: 2 out]
                    n107 = Number To Engineering String(2:i16 3 ("precision (6)"), 4:w369) -> (0:w371:string)  [unwired: 2 out]
                    n108 = Concatenate Strings(w360, "[var 1']") -> (w364:string)
                    n109 = Concatenate Strings("Offset: ", w372) -> (w367:string)
                    n110 = Concatenate Strings("Ratio: ", w371) -> (w366:string)
                  }
                  frame 4 {
                    w389 = ""
                    n111 = Unbundle By Name(w385) -> ("Mode"=w381:u32)
                    n112 = Unbundle By Name(w385) -> ("Start / Offset"=w391:dbl)
                    n113 = case shown="4, Default" w381 {
                      tunnel: ["Common" "Voltage Source " "Current Source " "Pulsed Voltage Source " "Pulsed Current Source "] -> w382
                      frame 4, Default {
                      }
                      frame 0 {
                      }
                      frame 1 {
                      }
                      frame 2 {
                      }
                      frame 3 {
                      }
                    }
                    n114 = Unbundle By Name(w385) -> ("Mode"=w388:u32)
                    n115 = case shown="0, 2, Default" w388 {
                      tunnel: [" V" " A"] -> w387
                      frame 0, 2, Default {
                      }
                      frame 1, 3 {
                      }
                    }
                    n116 = Number To Engineering String(2:i16 3 ("precision (6)"), 4:w391) -> (0:w393:string)  [unwired: 2 out]
                    n117 = Concatenate Strings("Value: ", w393, w387) -> (w386:string)
                    n118 = Concatenate Strings("Constant ", w382) -> (w384:string)
                  }
                }
                n119 = Equal To 0?(x=w276) -> (x = 0?=w275:bool)
                n120 = Unbundle By Name(w263) -> ("Compliance"=w279:dbl)
                n121 = Unbundle By Name(w263) -> ("Mode"=w284:u32)
                n122 = case shown="False" w275 {
                  tunnel: w276 -> [w405 _]
                  tunnel: [w402 "OFF"] -> w278
                  frame False {
                    n123 = Number To Engineering String(2:i16 3 ("precision (6)"), 4:w405) -> (0:w404:string)  [unwired: 2 out]
                    n124 = Concatenate Strings(w404, " W") -> (w402:string)
                  }
                  frame True {
                  }
                }
                n125 = case shown="0, 2, Default" w284 {
                  tunnel: [" A" " V"] -> w287
                  frame 0, 2, Default {
                  }
                  frame 1, 3 {
                  }
                }
                n126 = Number To Engineering String(2:i16 3 ("precision (6)"), 4:w279) -> (0:w286:string)  [unwired: 2 out]
                n127 = Concatenate Strings(w288, w289, ": ") -> (w272:string)
                n128 = Concatenate Strings("Compliance: ", w286, w287) -> (w267:string)
                n129 = Concatenate Strings("Power Compliance: ", w278) -> (w266:string)
                n130 = Concatenate Strings("Function: ", w282) -> (w271:string)
                n131 = Insert Into Array(array=w273, new element #1=w272, new element #2=w271, new element #3=w270, new element #4=w269, new element #5=w268, new element #6=w267, new element #7=w266, new element #8="\r") -> (w274:string[])  [unwired: 1 in]
              }
              n132 = Unbundle By Name(w227) -> ("Wait Time Parameter"=w235:dbl)
              n133 = Unbundle By Name(w227) -> ("Integration Time"=w228:u32)
              n134 = case "Sweep spacing" shown="1" w255 {
                tunnel: ["Linear" "Log 10" "Log 25" "Log 50"] -> w253
                frame 0, Default {
                  # "Linear"
                }
                frame 1 {
                  # "Log 10"
                }
                frame 2 {
                  # "Log 25"
                }
                frame 3 {
                  # "Log 50"
                }
              }
              n135 = case "Range" shown="0, Default" w252 {
                tunnel: ["Auto" "Fixed" "Limited"] -> w250
                frame 0, Default {
                }
                frame 1 {
                }
                frame 2 {
                }
              }
              n136 = case "Integration Time" shown="0, Default" w228 {
                tunnel: w227 -> [w258 w261]
                tunnel: [w257 w260] -> w229
                tunnel: ["Integration Time (Short): " "Integration Time (Long): "] -> w232
                frame 0, Default {
                  # "Short"
                  n137 = Unbundle By Name(w258) -> ("Short Integration Time (s)"=w257:dbl)
                }
                frame 1 {
                  # "Long"
                  n138 = Unbundle By Name(w261) -> ("Long Integration Time (s)"=w260:dbl)
                }
              }
              n139 = Number To Engineering String(2:i16 1 ("precision (6)"), 4:w235) -> (0:w237:string)  [unwired: 2 out]
              n140 = Concatenate Strings("Range: ", w250) -> (w240:string)
              n141 = Concatenate Strings("Sweep Spacing:  ", w253) -> (w241:string)
              n142 = Number To Engineering String(2:i16 5 ("precision (6)"), 3:i16 4 ("width (-)"), 4:w229) -> (0:w231:string)  [unwired: 1 out]
              n143 = Concatenate Strings(w232, w231, " s\n" ("string"), "Wait Time Parameter: ", w237) -> (w225:string)
              n144 = Insert Into Array(array=w242, new element #1=w241, new element #2=w240, new element #3=w225) -> (w239:string[])  [unwired: 1 in]
            }
            frame "Sampling Mode" {
              n145 = Unbundle By Name(w461) -> ("SMU1 - Sampling"=w466:T20, "SMU2 - Sampling"=w465:T20, "SMU3 - Sampling"=w464:T20, "SMU4 - Sampling"=w463:T20, "Sampling Time Parameters"=w436:T21, "Stop Condition"=w429:T22)
              n146 = Unbundle By Name(w436) -> ("Sampling Mode"=w455:i32, "Initial Interval (s)"=w456:dbl, "Number of Samples"=w457:i32, "Sampling Time"=w458:i32, "Hold Time (s)"=w459:dbl, "Total Sampling Time (s)"=w460:dbl)
              n147 = Unbundle By Name(w429) -> ("Stop Condition Enable"=w435:bool, "Name"=w434:string, "Event"=w433:i32, "Threshold"=w432:dbl, "num. of events"=w431:i32, "Enable Delay (s)"=w430:dbl)
              n148 = Build Array(w466, w465, w464, w463) -> (w462:T20[])
              n149 = for {
                shift-right: [w508] -> w428
                shift-left: string[] ["Sampling Acquisition Mode\n"] -> [w510]
                tunnel: "SMU" -> [w519]
                tunnel: w462 -> [w511] mode=indexing
                i -> [w518]
                n150 = Unbundle By Name(w511) -> ("Function"=w514:bool)
                n151 = Increment(x=w518) -> (x+1=w517:i32)
                n152 = Number To Decimal String(number=w517, width (-)=i16 1) -> (decimal integer string=w515:string)
                n153 = case shown="True" w514 {
                  tunnel: ["Disabled" w525] -> w512
                  tunnel: [w520 w524] -> w507
                  tunnel: [w520 w523] -> w506
                  tunnel: w511 -> [_ w522]
                  frame False {
                    w520 = ""
                  }
                  frame True {
                    n154 = Unbundle By Name(w522) -> ("Mode"=w528:u32, "Source"=w527:dbl, "Compliance"=w526:dbl)
                    n155 = case shown="2" w528 {
                      tunnel: ["Voltage Source" "Current Source" "Common"] -> w525
                      tunnel: w527 -> [w532 w553 _]
                      tunnel: w526 -> [w529 w550 _]
                      tunnel: [w531 w543 w555] -> w524
                      tunnel: [w530 w542 w555] -> w523
                      frame 0, Default {
                        n156 = Number To Engineering String(2:i16 3 ("precision (6)"), 4:w532) -> (0:w537:string)  [unwired: 2 out]
                        n157 = Number To Engineering String(2:i16 3 ("precision (6)"), 4:w529) -> (0:w534:string)  [unwired: 2 out]
                        n158 = Concatenate Strings("Value: ", w537, " V") -> (w531:string)
                        n159 = Concatenate Strings("Compliance: ", w534, " A") -> (w530:string)
                      }
                      frame 1 {
                        n160 = Number To Engineering String(2:i16 3 ("precision (6)"), 4:w553) -> (0:w548:string)  [unwired: 2 out]
                        n161 = Number To Engineering String(2:i16 3 ("precision (6)"), 4:w550) -> (0:w545:string)  [unwired: 2 out]
                        n162 = Concatenate Strings("Value: ", w548, " A") -> (w543:string)
                        n163 = Concatenate Strings("Compliance: ", w545, " V") -> (w542:string)
                      }
                      frame 2 {
                        w555 = ""
                      }
                    }
                  }
                }
                n164 = Concatenate Strings(w519, w515, ": ", w512) -> (w509:string)
                n165 = Insert Into Array(array=w510, new element #1=w509, new element #2=w507, new element #3=w506, new element #4="\r") -> (w508:string[])  [unwired: 1 in]
              }
              n166 = case shown="True" w435 {
                tunnel: ["Disabled" w480] -> w415
                tunnel: [w469 w479] -> w416
                tunnel: [w469 w478] -> w417
                tunnel: [w469 w477] -> w418
                tunnel: [w469 w476] -> w419
                tunnel: w434 -> [_ w475]
                tunnel: w433 -> [_ w474]
                tunnel: w432 -> [_ w473]
                tunnel: w431 -> [_ w472]
                tunnel: w430 -> [_ w471]
                frame False {
                  w469 = ""
                }
                frame True {
                  n167 = case shown="2" w474 {
                    tunnel: ["Value > Threshold" "Value < Threshold" "| Value | > | Threshold |" "| Value | < | Threshold |"] -> w491
                    frame 0, Default {
                    }
                    frame 1 {
                    }
                    frame 2 {
                    }
                    frame 3 {
                    }
                  }
                  n168 = Number To Engineering String(2:i16 3 ("precision (6)"), 4:w473) -> (0:w489:string)  [unwired: 2 out]
                  n169 = Number To Decimal String(number=w472) -> (decimal integer string=w486:string)  [unwired: 1 out]
                  n170 = Number To Engineering String(2:i16 3 ("precision (6)"), 4:w471) -> (0:w484:string)  [unwired: 2 out]
                  n171 = Concatenate Strings("Name: ", w475) -> (w480:string)
                  n172 = Concatenate Strings("Event type: ", w491) -> (w479:string)
                  n173 = Concatenate Strings("Number of Events: ", w486) -> (w477:string)
                  n174 = Concatenate Strings("Threshold: ", w489) -> (w478:string)
                  n175 = Concatenate Strings("Enable Delay: ", w484, " s") -> (w476:string)
                }
              }
              n176 = Number To Engineering String(2:i16 3 ("precision (6)"), 4:w460) -> (0:w447:string)  [unwired: 2 out]
              n177 = case shown="4" w455 {
                tunnel: ["Linear" "Log 10" "Log 25" "Log 50" "Thinend Out"] -> w441
                frame 0, Default {
                }
                frame 1 {
                }
                frame 2 {
                }
                frame 3 {
                }
                frame 4 {
                }
              }
              n178 = case shown="0, Default" w458 {
                tunnel: ["Auto (linear only)" "No Limit" "Set Limit"] -> w453
                frame 0, Default {
                }
                frame 1 {
                }
                frame 2 {
                }
              }
              n179 = Number To Engineering String(2:i16 3 ("precision (6)"), 4:w456) -> (0:w445:string)  [unwired: 2 out]
              n180 = Number To Decimal String(number=w457) -> (decimal integer string=w452:string)  [unwired: 1 out]
              n181 = Number To Engineering String(2:i16 3 ("precision (6)"), 4:w459) -> (0:w451:string)  [unwired: 2 out]
              n182 = Concatenate Strings("Sampling Mode: ", w441) -> (w425:string)
              n183 = Concatenate Strings("Initial Interval: ", w445, " s") -> (w424:string)
              n184 = Concatenate Strings("Number of Samples: ", w452) -> (w423:string)
              n185 = Concatenate Strings("Sampling Time: ", w453) -> (w422:string)
              n186 = Concatenate Strings("Hold Time: ", w451, " s") -> (w421:string)
              n187 = Concatenate Strings("Total Sampling Time: ", w447, " s") -> (w420:string)
              n188 = Insert Into Array(array=w428, new element #1="\nSampling Parameters:\n", new element #2=w425, new element #3=w424, new element #4=w423, new element #5=w422, new element #6=w421, new element #7=w420, new element #8="\nStop Condition:\n", new element #9=w415, new element #10=w416, new element #11=w417, new element #12=w418, new element #13=w419) -> (w427:string[])  [unwired: 1 in]
            }
          }
          n189 = for "Concatenate Strings with CR/LF" {
            shift-right: [w558] -> w221
            shift-left: "" -> [w560]
            tunnel: "\n" ("string") -> [w559]
            tunnel: w218 -> [w557] mode=indexing
            n190 = case "With the exeption of \nempty strings" shown="Default" w557 {
              selector: w557 -> [_ w562]
              tunnel: w560 -> [w561 w565]
              tunnel: w559 -> [_ w564]
              tunnel: [w561 w563] -> w558
              frame "" {
              }
              frame Default {
                n191 = Concatenate Strings(w565, w562, w564) -> (w563:string)
              }
            }
          }
        }
        frame Error {
        }
      }
      n192 = Bundle By Name(cluster=T1 {"Instrument"=enum."Parameter Analyzer", "Configuration"="Test Configuration"} ("Instrument Configuration 2"), "Configuration"=w210) -> (w208:T1)
    }
    frame "Unknown Instrument", Default {
      n193 = call "Dialog.vi"("error in (no error)"=w570, "message"="Cannot Convert Configuration into String: Unknown Instrument") -> ("error out"=w571:errorcluster)  [unwired: 1 in, 8 out]
    }
  }
  "error out" <- w2
  "Instrument Configuration" <- w1
